vi "Read Four Shim Pision.vi"(11 "Value":string[](array[string])) -> (0 "点位":cluster{"X":dbl, "Y":dbl, "Z":dbl, "U":dbl}[](array[cluster]), 1 "三点位置":dbl[][](array[numeric]), 2 "列":i32, 3 "行":i32)   [LabVIEW 2011]
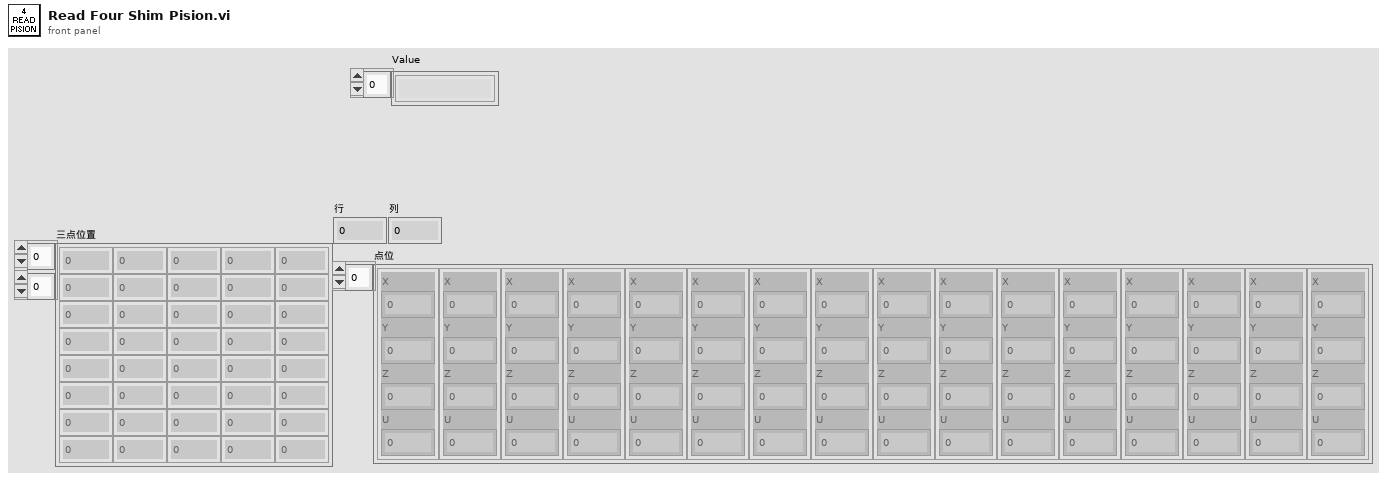
[diagram p1: front panel]
types:
  T1 = cluster{"String in":string, "String in":string, "String in":string, "String in":string}
  T2 = cluster{"String in":dbl, "String in":dbl, "String in":dbl, "String in":dbl}[]
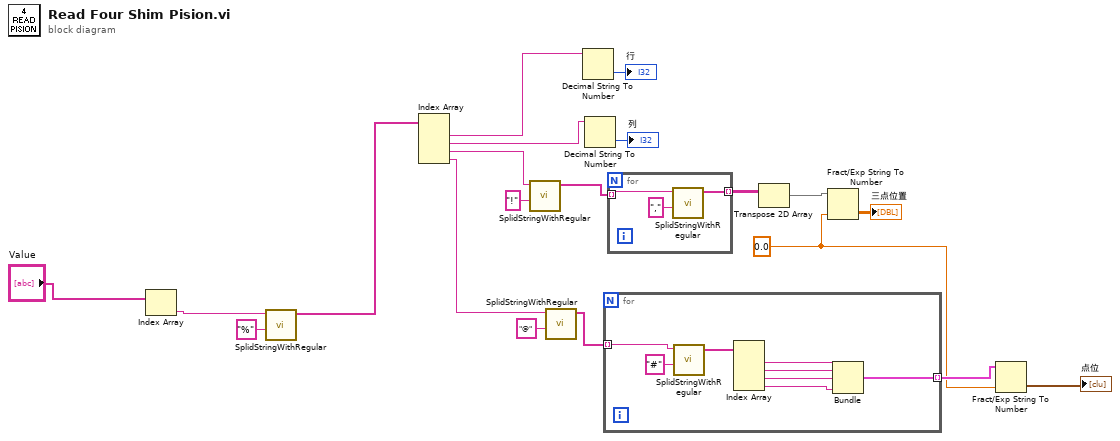
[diagram p0: block diagram]
diagram:
  w4 = 0.0
  n1 = Index Array(array="Value") -> (element=w1:string)  [unwired: 1 in]
  n2 = call "SplidStringWithRegular.vi"("regular expression"="%", "String in"=w1) -> ("Array out"=w19:string[])  [unwired: 9 in]
  n3 = Index Array(array=w19) -> (element #1=w18:string, element #2=w17:string, element #3=w16:string, element #4=w7:string)  [unwired: 4 in]
  n4 = call "SplidStringWithRegular.vi"("regular expression"="!", "String in"=w16) -> ("Array out"=w14:string[])  [unwired: 9 in]
  n5 = call "SplidStringWithRegular.vi"("regular expression"="@", "String in"=w7) -> ("Array out"=w6:string[])  [unwired: 9 in]
  n6 = Decimal String To Number(string=w18) -> (number=→"行":i32)  [unwired: 2 in, 1 out]
  n7 = Decimal String To Number(string=w17) -> (number=→"列":i32)  [unwired: 2 in, 1 out]
  n8 = for {
    tunnel: w6 -> [w27] mode=indexing
    tunnel: [w21] -> w5 mode=indexing
    n9 = call "SplidStringWithRegular.vi"("regular expression"="#", "String in"=w27) -> ("Array out"=w26:string[])  [unwired: 9 in]
    n10 = Index Array(array=w26) -> (element #1=w25:string, element #2=w24:string, element #3=w23:string, element #4=w22:string)  [unwired: 4 in]
    n11 = Bundle("String in"=w25, "String in"=w24, "String in"=w23, "String in"=w22) -> (w21:T1)  [unwired: 1 in]
  }
  n12 = for {
    tunnel: w14 -> [w31] mode=indexing
    tunnel: [w29] -> w13 mode=indexing
    n13 = call "SplidStringWithRegular.vi"("regular expression"=",", "String in"=w31) -> ("Array out"=w29:string[])  [unwired: 9 in]
  }
  n14 = Transpose 2D Array(2D array=w13) -> (transposed array=w12:string[][])
  n15 = Fract/Exp String To Number(string=w12, default (0 dbl)=w4) -> (number=→"三点位置":dbl[][])  [unwired: 2 in, 1 out]
  n16 = Fract/Exp String To Number(string=w5, default (0 dbl)=w4) -> (number=→"点位":T2)  [unwired: 2 in, 1 out]
